vi "OpenConnection.vi"(8 "error in (no error)":errorcluster, 11 "object in":refnum<class "TCP.lvclass">) -> (0 "error out":errorcluster, 3 "object out":refnum<class "TCP.lvclass">)   [LabVIEW 2019, in "TCP.lvclass"]
uses:
  TCP.lvclass
  TCP.lvclass/TCP.ctl
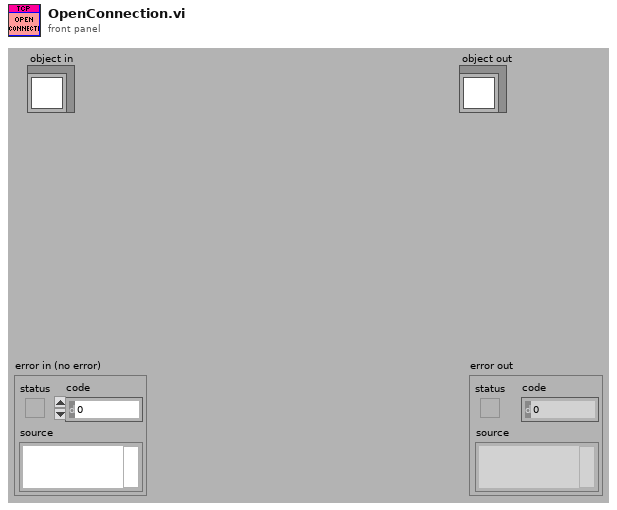
[diagram p1: front panel]
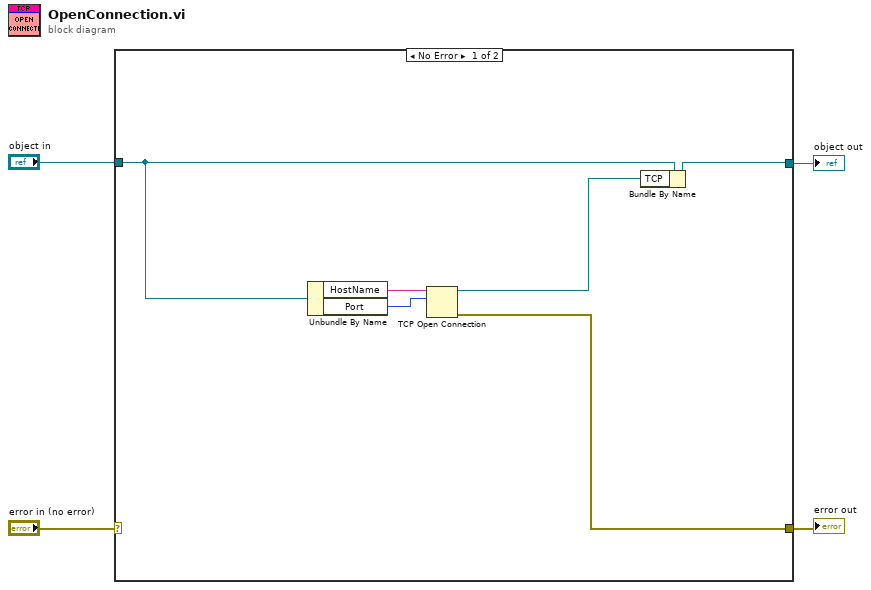
[diagram p0: block diagram]
diagram:
  n1 = case shown="No Error" "error in (no error)" {
    selector: "error in (no error)" -> [_ w12]
    tunnel: [w7 w12] -> w3
    tunnel: [w6 w11] -> w1
    tunnel: "object in" -> [w10 w11]
    frame No Error {
      n2 = Unbundle By Name(w10) -> ("HostName"=w9:string, "Port"=w8:u16)
      n3 = TCP Open Connection(address=w9, remote port or service name=w8) -> (connection ID=w5:refnum<k5>, error out=w7:errorcluster)  [unwired: 3 in]
      n4 = Bundle By Name(cluster=w10, "TCP"=w5) -> (w6:refnum<class "TCP.lvclass">)
    }
    frame Error {
    }
  }
  "error out" <- w3
  "object out" <- w1
